vi "FIFO Flush.vi"(8 "Error In":errorcluster, 10 "Logging queue element in":T1 {"Ref Dwell time (us)" format="%#.6g"; "Frame Size" items=["100X100"=100, "128X128"=128, "200X200"=200, "256X256"=256, "512X512"=512, "1024x1024"=1024, "2048x2048"=2048]; "Dwell time (us)" format="%#.6g"}, 11 "FPGA VI Ref":T5) -> (0 "Error Out":errorcluster, 2 "Ch0 Elements Remaining":u32, 3 "FPGA VI Reference Out":T5)   [LabVIEW 2020]
uses:
  RIG-SPECIFIC FILES/FPGA Refs/FPGA Ref.ctl
  Typedefs/Logging queue element.ctl
  Typedefs/Imaging Protocols enum.ctl
  Typedefs/Frame Size.ctl
  Typedefs/Acquired points count.ctl
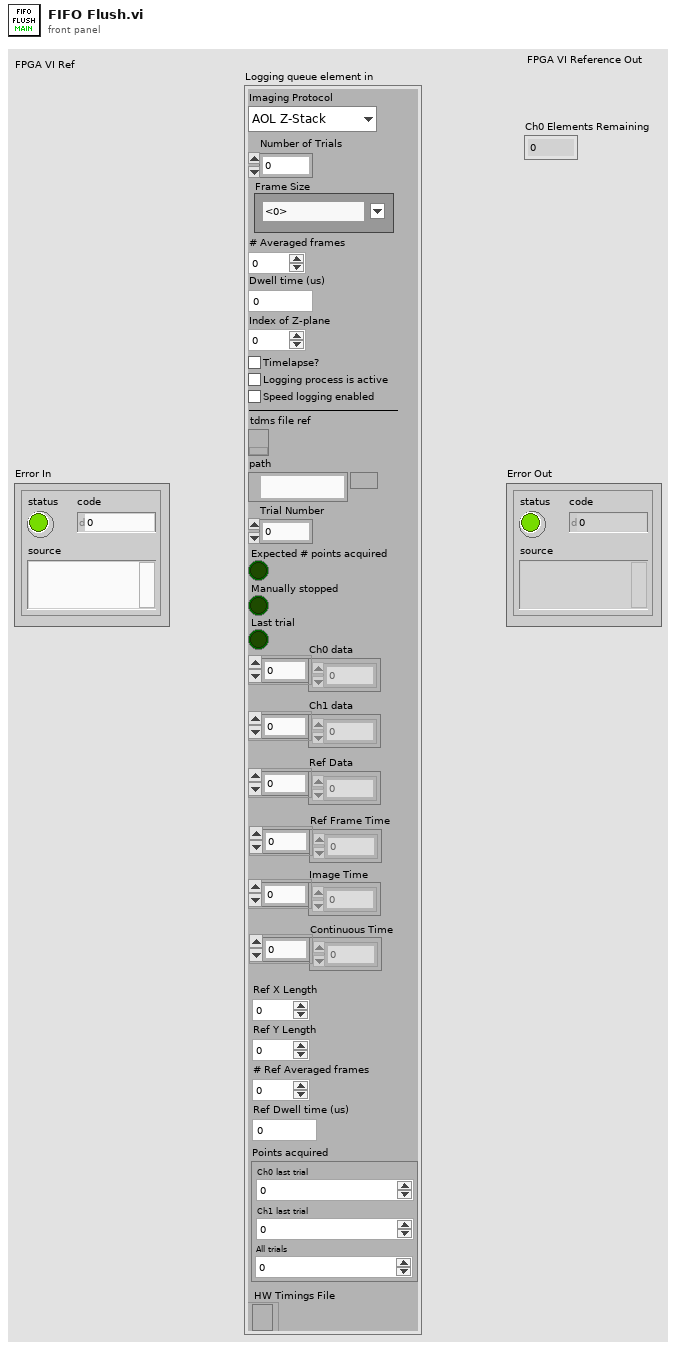
[diagram p1: front panel]
types:
  T1 = typedef "Logging queue element.ctl" = cluster{"Imaging Protocol":T2, "Number of Trials":u16, "Frame Size":T3, "# Averaged frames":u16, "Dwell time (us)":dbl, "Index of Z-plane":i32, "Timelapse?":bool, "Logging process is active":bool, "Speed logging enabled":bool, "tdms file ref":refnum<k34>, "path":path, "Trial Number":i32, "Expected # points acquired":bool, "Manually stopped":bool, "Last trial":bool, "Ch0 data":u32[], "Ch1 data":u32[], "Ref Data":u32[], "Ref Frame Time":u64[], "Image Time":u64[], "Continuous Time":u64[], "Ref X Length":u16, "Ref Y Length":u16, "# Ref Averaged frames":u16, "Ref Dwell time (us)":dbl, "Points acquired":T4, "HW Timings File":refnum<file>}
  T2 = typedef "Imaging Protocols enum.ctl" = enum16{"AOL Z-Stack", "Motor Z Stack", "Parameter Sweep", "Functional Acquisition", "Single Plane Acquisition", "Volume Acquisition", "Live Imaging", "Live Plane Imaging", "Live Volume Imaging"}
  T3 = typedef "Frame Size.ctl" = u16
  T4 = typedef "Acquired points count.ctl" = cluster{"Ch0 last trial":u64, "Ch1 last trial":u64, "All trials":u64}
  T5 = typedef "FPGA Ref.ctl" = refnum<k20>
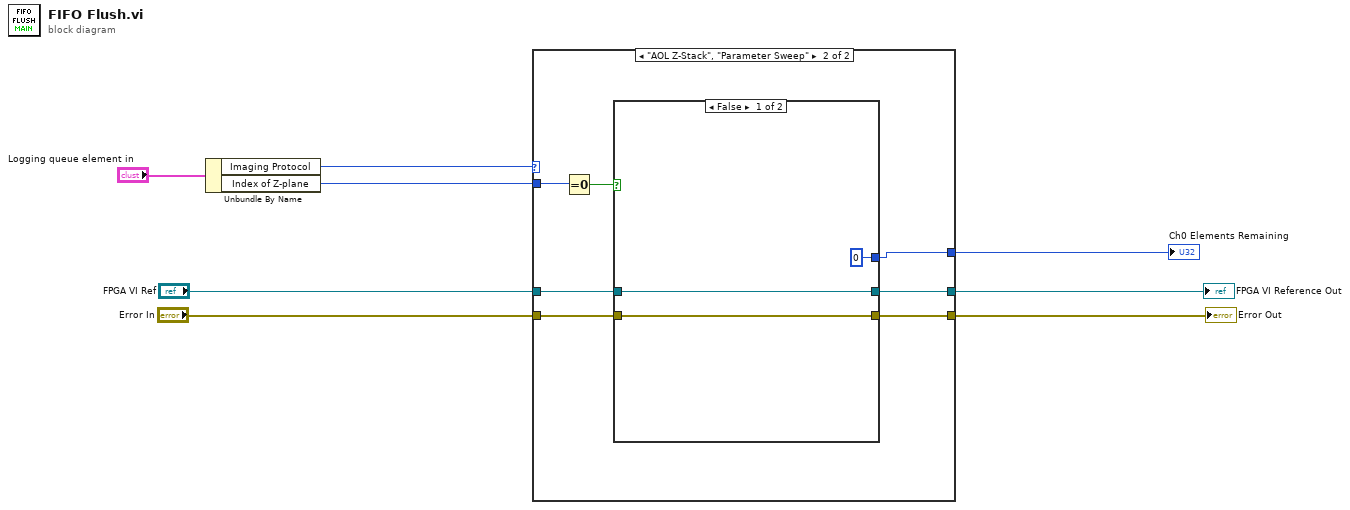
[diagram p0: block diagram]
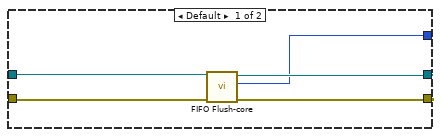
[diagram p2: hidden frame]
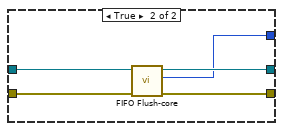
[diagram p3: hidden frame]
diagram:
  n1 = Unbundle By Name("Logging queue element in") -> ("Imaging Protocol"=w3:T2, "Index of Z-plane"=w1:i32)
  n2 = case shown="\"AOL Z-Stack\", \"Parameter Sweep\"" w3 {
    tunnel: "FPGA VI Ref" -> [w13 w20]
    tunnel: "Error In" -> [w12 w19]
    tunnel: [w11 w18] -> w6
    tunnel: [w10 w17] -> w5
    tunnel: [w9 w16] -> w2
    tunnel: w1 -> [_ w15]
    frame Default {
      n3 = call "FIFO Flush-core.vi"("Error In"=w12, "FPGA VI Ref"=w13) -> ("Error Out"=w10:errorcluster, "Ch0 Elements Remaining"=w9:u32, "FPGA VI Reference Out"=w11:T5)  [unwired: 7 in]
    }
    frame "AOL Z-Stack", "Parameter Sweep" {
      n4 = Equal To 0?(x=w15) -> (x = 0?=w14:bool)
      n5 = case shown="False" w14 {
        tunnel: w20 -> [w22 w28]
        tunnel: w19 -> [w23 w27]
        tunnel: [w22 w26] -> w18
        tunnel: [w23 w25] -> w17
        tunnel: [u32 0 ("Ch0 Elements Remaining") w24] -> w16
        frame False {
        }
        frame True {
          n6 = call "FIFO Flush-core.vi"("Error In"=w27, "FPGA VI Ref"=w28) -> ("Error Out"=w25:errorcluster, "Ch0 Elements Remaining"=w24:u32, "FPGA VI Reference Out"=w26:T5)  [unwired: 7 in]
        }
      }
    }
  }
  "FPGA VI Reference Out" <- w6
  "Error Out" <- w5
  "Ch0 Elements Remaining" <- w2
